vi "Configure Measurement Signal.vi"(7 "Signal Frequency (1000 Hz)":dbl=1000.0, 8 "error in (no error)":errorcluster, 9 "Signal Level (1.0 V)":dbl=1.0, 10 "Signal Type (0: Voltage)":u16(ring) items=["Voltage", "Current"], 11 "VISA resource name":refnum<visa-resource-name>) -> (0 "error out":errorcluster, 3 "VISA resource name out":refnum<visa-resource-name>)   [LabVIEW 2017, in "Agilent E4980.lvlib"]
doc: "Sets the oscillator output signal frequency and level. You can set the oscillator level as appropriate voltage or current value.\n\n<B>Notes:</B>\n(1) By using the automatic level control (ALC) function, the actual signal level applied to the DUT can be the same as the setting value."
uses:
  Agilent E4980.lvlib
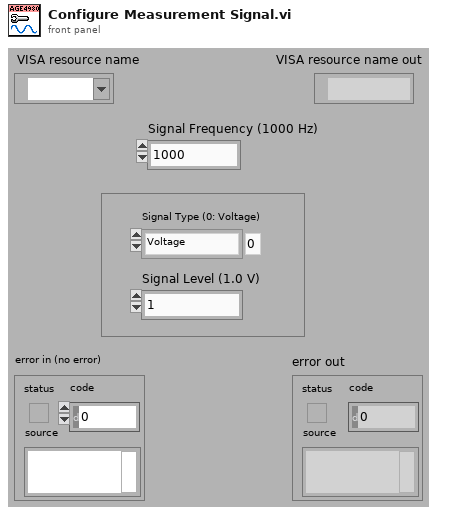
[diagram p1: front panel]
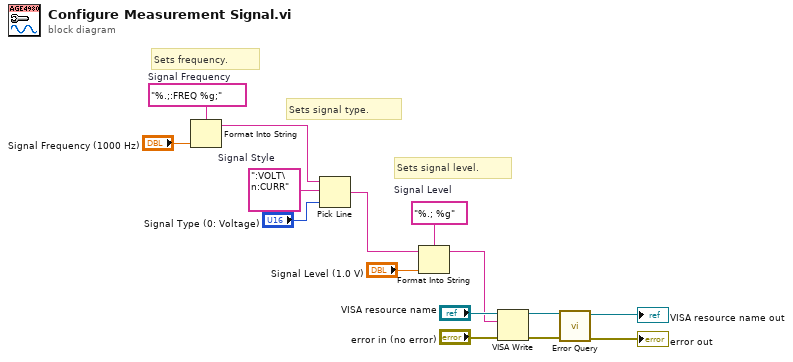
[diagram p0: block diagram]
diagram:
  w8 = "%.; %g"  # Signal Level
  w10 = ":VOLT\n:CURR"  # Signal Style
  w14 = "%.;:FREQ %g;"  # Signal Frequency
  # "Sets signal level."
  # "Sets signal type."
  # "Sets frequency."
  n1 = Format Into String(format string=w14, "Signal Frequency (1000 Hz)") -> (resulting string=w1:string)  [unwired: 2 in, 1 out]
  n2 = Pick Line(string ("")=w1, multi-line string=w10, line index="Signal Type (0: Voltage)") -> (output string=w9:string)
  n3 = Format Into String(format string=w8, initial string=w9, "Signal Level (1.0 V)") -> (resulting string=w6:string)  [unwired: 1 in, 1 out]
  n4 = VISA Write(VISA resource name="VISA resource name", write buffer=w6, error in (no error)="error in (no error)") -> (VISA resource name out=w5:refnum<visa-resource-name>, error out=w4:errorcluster)  [unwired: 1 out]
  n5 = call "Error Query.vi"("error in (no error)"=w4, "VISA resource name"=w5) -> ("error out"=→"error out":errorcluster, "VISA resource name out"=→"VISA resource name out":refnum<visa-resource-name>)  [unwired: 6 in, 2 out]
